vi "FFT Measurement Test UI.vi"() -> ()   [LabVIEW 2014]
uses:
  <vilib>/rvi/interface/RandomDataEmulation/nirviRandomDataOpen.vi
  <vilib>/rvi/interface/common/niFpgaCacheSessionInfoDynamic.vi
  <vilib>/rvi/interface/common/niFpgaWaitOnOcc.vi
  <vilib>/Utility/error.llb/Error Cluster From Error Code.vi
  <vilib>/rvi/errors/niLvFpgaAdjustHostInterfaceError.vi
  <vilib>/FPGAPlugInAG/Dynamic/niLvFpga_Close_Dynamic.vi
  <vilib>/rvi/interface/nirviOpenFPGA/nirviOpenFPGA.xnode
  FPGA Target/Test VIs/FFT Simulation test.vi
  <vilib>/rvi/interface/nirviMethod/nirviMethod.xnode
  <vilib>/rvi/interface/nirviCloseFPGA/nirviCloseFPGA.xnode
  <vilib>/FPGAPlugInAG/Dynamic/niLvFpga_ConfigureFifo_Dynamic.vi
  <vilib>/rvi/errors/niLvFpgaMergeErrorWithErrorCode.vi
  <vilib>/FPGAPlugInAG/Dynamic/niLvFpga_StartFifo_Dynamic.vi
  <vilib>/FPGAPlugInAG/Dynamic/niLvFpga_ReadFifo_Dynamic.vi
  <vilib>/rvi/Analysis/host/Public/NI_FpgaMspHost.lvlib
panel:
  out "Error %":dbl
  out "Theoretical Freq.":dbl
  in  "#Periods":dbl=1.0
  in  "#Samples":dbl=1.0
  in  "Gen. Freq.":dbl=1.0
  out "Waveform Graph":dbl[](graph)
  out "Detected Frequency (Hz)":dbl
  out "Index Bin":dbl
  out "Signal":waveform(dbl)(graph)
  # "Theoretical Results"
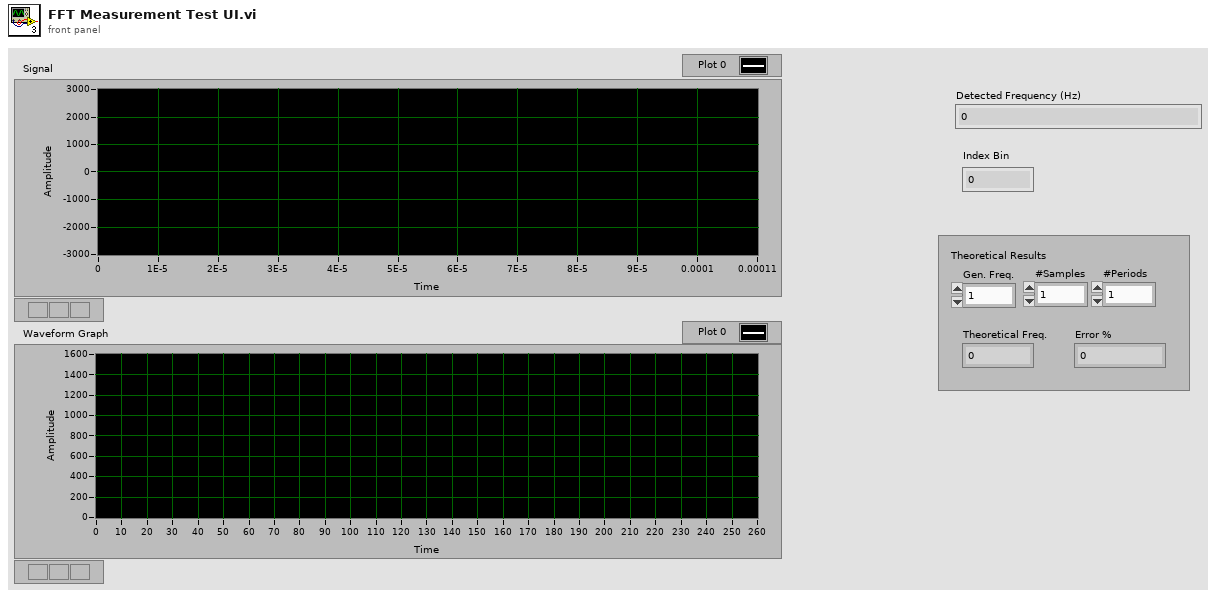
[diagram p1: front panel]
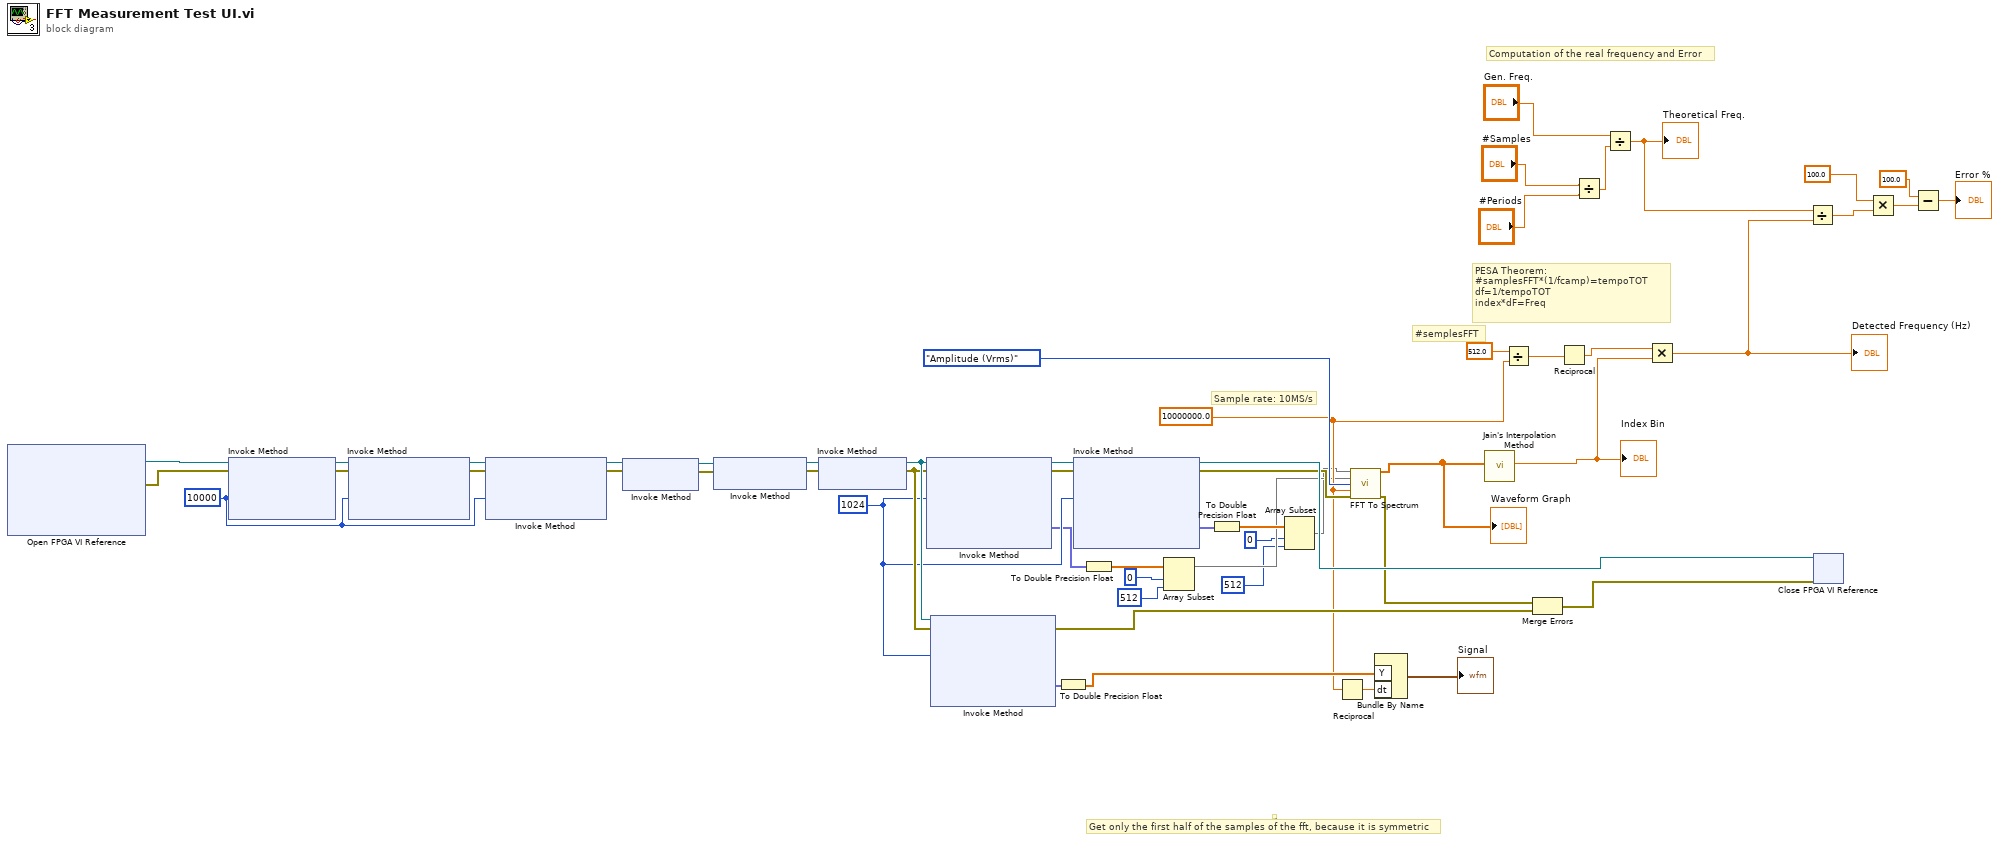
[diagram p0: block diagram]
diagram:
  w23 = 10000000.0 ("Sample Rate (S/s)")
  w38 = u32 1024 ("Requested Depth")
  w51 = u32 10000 ("Requested Depth")
  # "Computation of the real frequency and Error"
  # "."
  # "Get only the first half of the samples of the fft, because it is symmetric"
  # "#semplesFFT"
  # "PESA Theorem:\n#samplesFFT*(1/fcamp)=tempoTOT\ndf=1/tempoTOT\nindex*dF=Freq"
  # "Sample rate: 10MS/s"
  n1 = xnode "Open FPGA VI Reference"() -> ("FPGA VI Reference Out"=w25:refnum<k20>, "error out"=w24:errorcluster)  [unwired: 2 in]
  n2 = xnode "Invoke Method"("FPGA VI Reference In"=w25, "error in"=w24, "Requested Depth"=w51) -> ("FPGA VI Reference Out"=w53:refnum<k20>, "error out"=w52:errorcluster)  [unwired: 1 out]
  n3 = xnode "Invoke Method"("FPGA VI Reference In"=w53, "error in"=w52, "Requested Depth"=w51) -> ("FPGA VI Reference Out"=w50:refnum<k20>, "error out"=w49:errorcluster)  [unwired: 1 out]
  n4 = xnode "Invoke Method"("FPGA VI Reference In"=w50, "error in"=w49, "Requested Depth"=w51) -> ("FPGA VI Reference Out"=w48:refnum<k20>, "error out"=w47:errorcluster)  [unwired: 1 out]
  n5 = xnode "Invoke Method"("FPGA VI Reference In"=w48, "error in"=w47) -> ("FPGA VI Reference Out"=w46:refnum<k20>, "error out"=w45:errorcluster)
  n6 = xnode "Invoke Method"("FPGA VI Reference In"=w46, "error in"=w45) -> ("FPGA VI Reference Out"=w41:refnum<k20>, "error out"=w44:errorcluster)
  n7 = xnode "Invoke Method"("FPGA VI Reference In"=w41, "error in"=w44) -> ("FPGA VI Reference Out"=w40:refnum<k20>, "error out"=w39:errorcluster)
  n8 = xnode "Invoke Method"("FPGA VI Reference In"=w40, "error in"=w39, "Number of Elements"=w38) -> ("FPGA VI Reference Out"=w43:refnum<k20>, "error out"=w42:errorcluster, "Data"=w30:fxp<+/-,22,22>[])  [unwired: 1 in, 1 out]
  n9 = xnode "Invoke Method"("FPGA VI Reference In"=w40, "error in"=w39, "Number of Elements"=w38) -> ("error out"=w26:errorcluster, "Data"=w37:fxp<+/-,12,12>[])  [unwired: 1 in, 2 out]
  n10 = To Double Precision Float(number=w37) -> (double precision float=w35:dbl[])
  n11 = xnode "Invoke Method"("FPGA VI Reference In"=w43, "error in"=w42, "Number of Elements"=w38) -> ("FPGA VI Reference Out"=w55:refnum<k20>, "error out"=w33:errorcluster, "Data"=w31:fxp<+/-,22,22>[])  [unwired: 1 in, 1 out]
  n12 = To Double Precision Float(number=w30) -> (double precision float=w28:dbl[])
  n13 = Array Subset(array=w28, index=0, length=512) -> (w17:dbl[])
  n14 = To Double Precision Float(number=w31) -> (double precision float=w29:dbl[])
  n15 = Array Subset(array=w29, index=0, length=512) -> (w14:dbl[])
  n16 = Reciprocal(x=w23) -> (1/x=w34:dbl)
  n17 = call <vilib>:"FFT To Spectrum.vi"("real FFT data"=w14, "imaginary FFT data"=w17, "spectrum type"=enum8{"Power (Vrms^2)", "Amplitude (Vrms)"}."Amplitude (Vrms)", "sample rate (S/s)"=w23, "error in (no error)"=w33) -> ("spectrum out"=w18:dbl[], "error out"=w32:errorcluster)  [unwired: 8 in, 1 out]
  "Waveform Graph" <- w18
  n18 = Bundle By Name("Y"=w35, "dt"=w34) -> (→"Signal":waveform(dbl))  [unwired: 1 in]
  n19 = call "Jain's Interpolation Method.vi"("FFT array"=w18) -> ("Index Bin"=w20:dbl)  [unwired: 9 in, 1 out]
  "Index Bin" <- w20
  n20 = Divide(x=512.0, y=w23) -> (x/y=w21:dbl)
  n21 = Merge Errors(w32, w26) -> (w54:errorcluster)
  n22 = Reciprocal(x=w21) -> (1/x=w19:dbl)
  n23 = Divide(x="#Samples", y="#Periods") -> (x/y=w11:dbl)
  n24 = Divide(x="Gen. Freq.", y=w11) -> (x/y=w8:dbl)
  "Theoretical Freq." <- w8
  n25 = Multiply(x=w19, y=w20) -> (x*y=w9:dbl)
  "Detected Frequency (Hz)" <- w9
  n26 = Divide(x=w8, y=w9) -> (x/y=w7:dbl)
  n27 = xnode "Close FPGA VI Reference"("FPGA VI Reference In"=w55, "error in"=w54) -> ()  [unwired: 1 out]
  n28 = Multiply(x=100.0, y=w7) -> (x*y=w3:dbl)
  n29 = Subtract(x=100.0, y=w3) -> (x-y=→"Error %":dbl)
